vi "FTW-TestExecutive-Core_StepTypes_Definitions.vi"(0 "FTW-CustomTestExecutive-Core In":refnum<class "FTW-CustomTestExecutive-Core.lvclass">, 11 "error in":errorcluster) -> (4 "FTW-CustomTestExecutive-Core Out":refnum<class "FTW-CustomTestExecutive-Core.lvclass">, 8 "Step Types":cluster{"Name":string, "Base Config":string}[](array[cluster]), 15 "error out":errorcluster)   [LabVIEW 2015, in "FTW-CustomTestExecutive-Core.lvclass"]
uses:
  FTW-CustomTestExecutive-Core.lvclass
  Test Steps/Wait/FTW-TestStep-Wait-Core.lvclass
  Test Steps/Wait/FTW-TestStep-Wait-Core_Step.vi
  Test Executive/core/FTW-TestExecutive-Core.lvclass
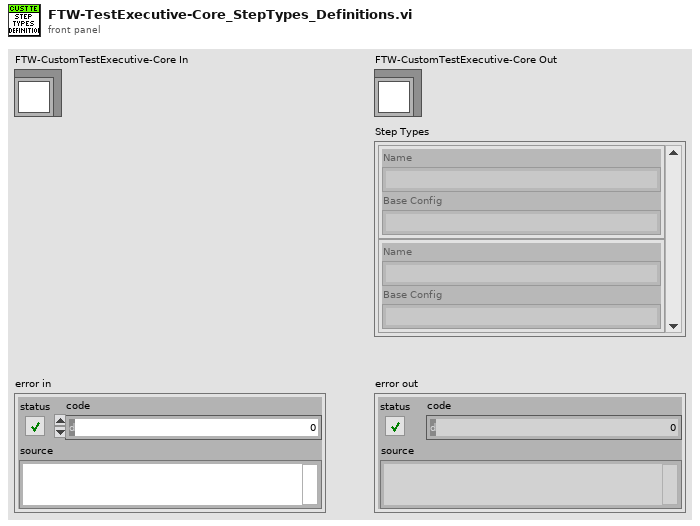
[diagram p1: front panel]
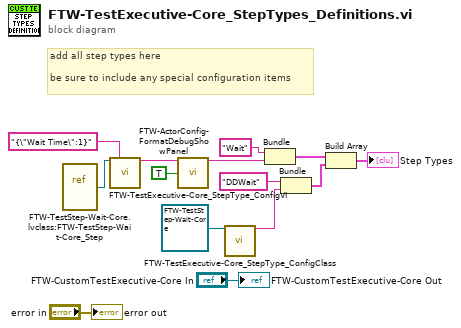
[diagram p0: block diagram]
diagram:
  # "add all step types here\n\nbe sure to include any special configuration items"
  n1 = vi-ref "FTW-TestStep-Wait-Core.lvclass:FTW-TestStep-Wait-Core_Step.vi"() -> (w12:refnum<vi>)
  n2 = call "FTW-TestExecutive-Core_StepType_ConfigVI.vi"("Step Actor"=w12, "Other Config Items"="{\"Wait Time\":1}") -> ("Base Config String"=w14:string)  [unwired: 13 in]
  n3 = call "FTW-ActorConfig-FormatDebugShowPanel.vi"("FTW Config String In"=w14, "Show Panel"=TRUE) -> ("FTW Config String"=w6:string)  [unwired: 12 in, 1 out]
  n4 = call "FTW-TestExecutive-Core_StepType_ConfigClass.vi"("Step Class"=refnum<class "FTW-TestStep-Wait-Core.lvclass"> refnum ("FTW-TestStep-Wait-Core")) -> ("Base Config String"=w3:string)  [unwired: 14 in]
  n5 = Bundle("Wait", "FTW Config String"=w6) -> (w11:cluster{string, "FTW Config String":string})  [unwired: 1 in]
  n6 = Bundle("DDWait", "Base Config String"=w3) -> (w1:cluster{string, "Base Config String":string})  [unwired: 1 in]
  n7 = Build Array(w11, w1) -> (→"Step Types":cluster{string, "Base Config String":string}[])
  "FTW-CustomTestExecutive-Core Out" <- "FTW-CustomTestExecutive-Core In"
  "error out" <- "error in"
